vi "Ionospheric image processing ver.1.0 .vi"() -> ()   [LabVIEW 2021]
panel:
  in  "新元素/子数组":i32=1
  out "骨骼化1":dbl[][](graph)
  out "腐蚀":dbl[][](graph)
  out "膨胀":dbl[][](graph)
  out "强度图":dbl[][](graph)
  out "大小":i32[](array[numeric])
  in  "y":i32
  out "x与y？":bool
  out "骨骼化0.5":dbl[][](graph)
  in  "dy":dbl=2.5 format="%#_13g"
  in  "y_max":dbl=900.0 format="%#_13g"
  in  "y_min":dbl format="%#_13g"
  in  "dx":dbl=0.05 format="%#_13g"
  in  "x_max":dbl=10.0 format="%#_13g"
  in  "x_min":dbl=1.5 format="%#_13g"
  in  "路径":path
  # "x:1.5-10\ny:0-900\ndx:0.05\ndy:2.5"
  # "每个x对应多个y值，取中位数或平均值，同时参考x前的值或x后的值，使得曲线变得更加平滑\n（需了解相关函数）"
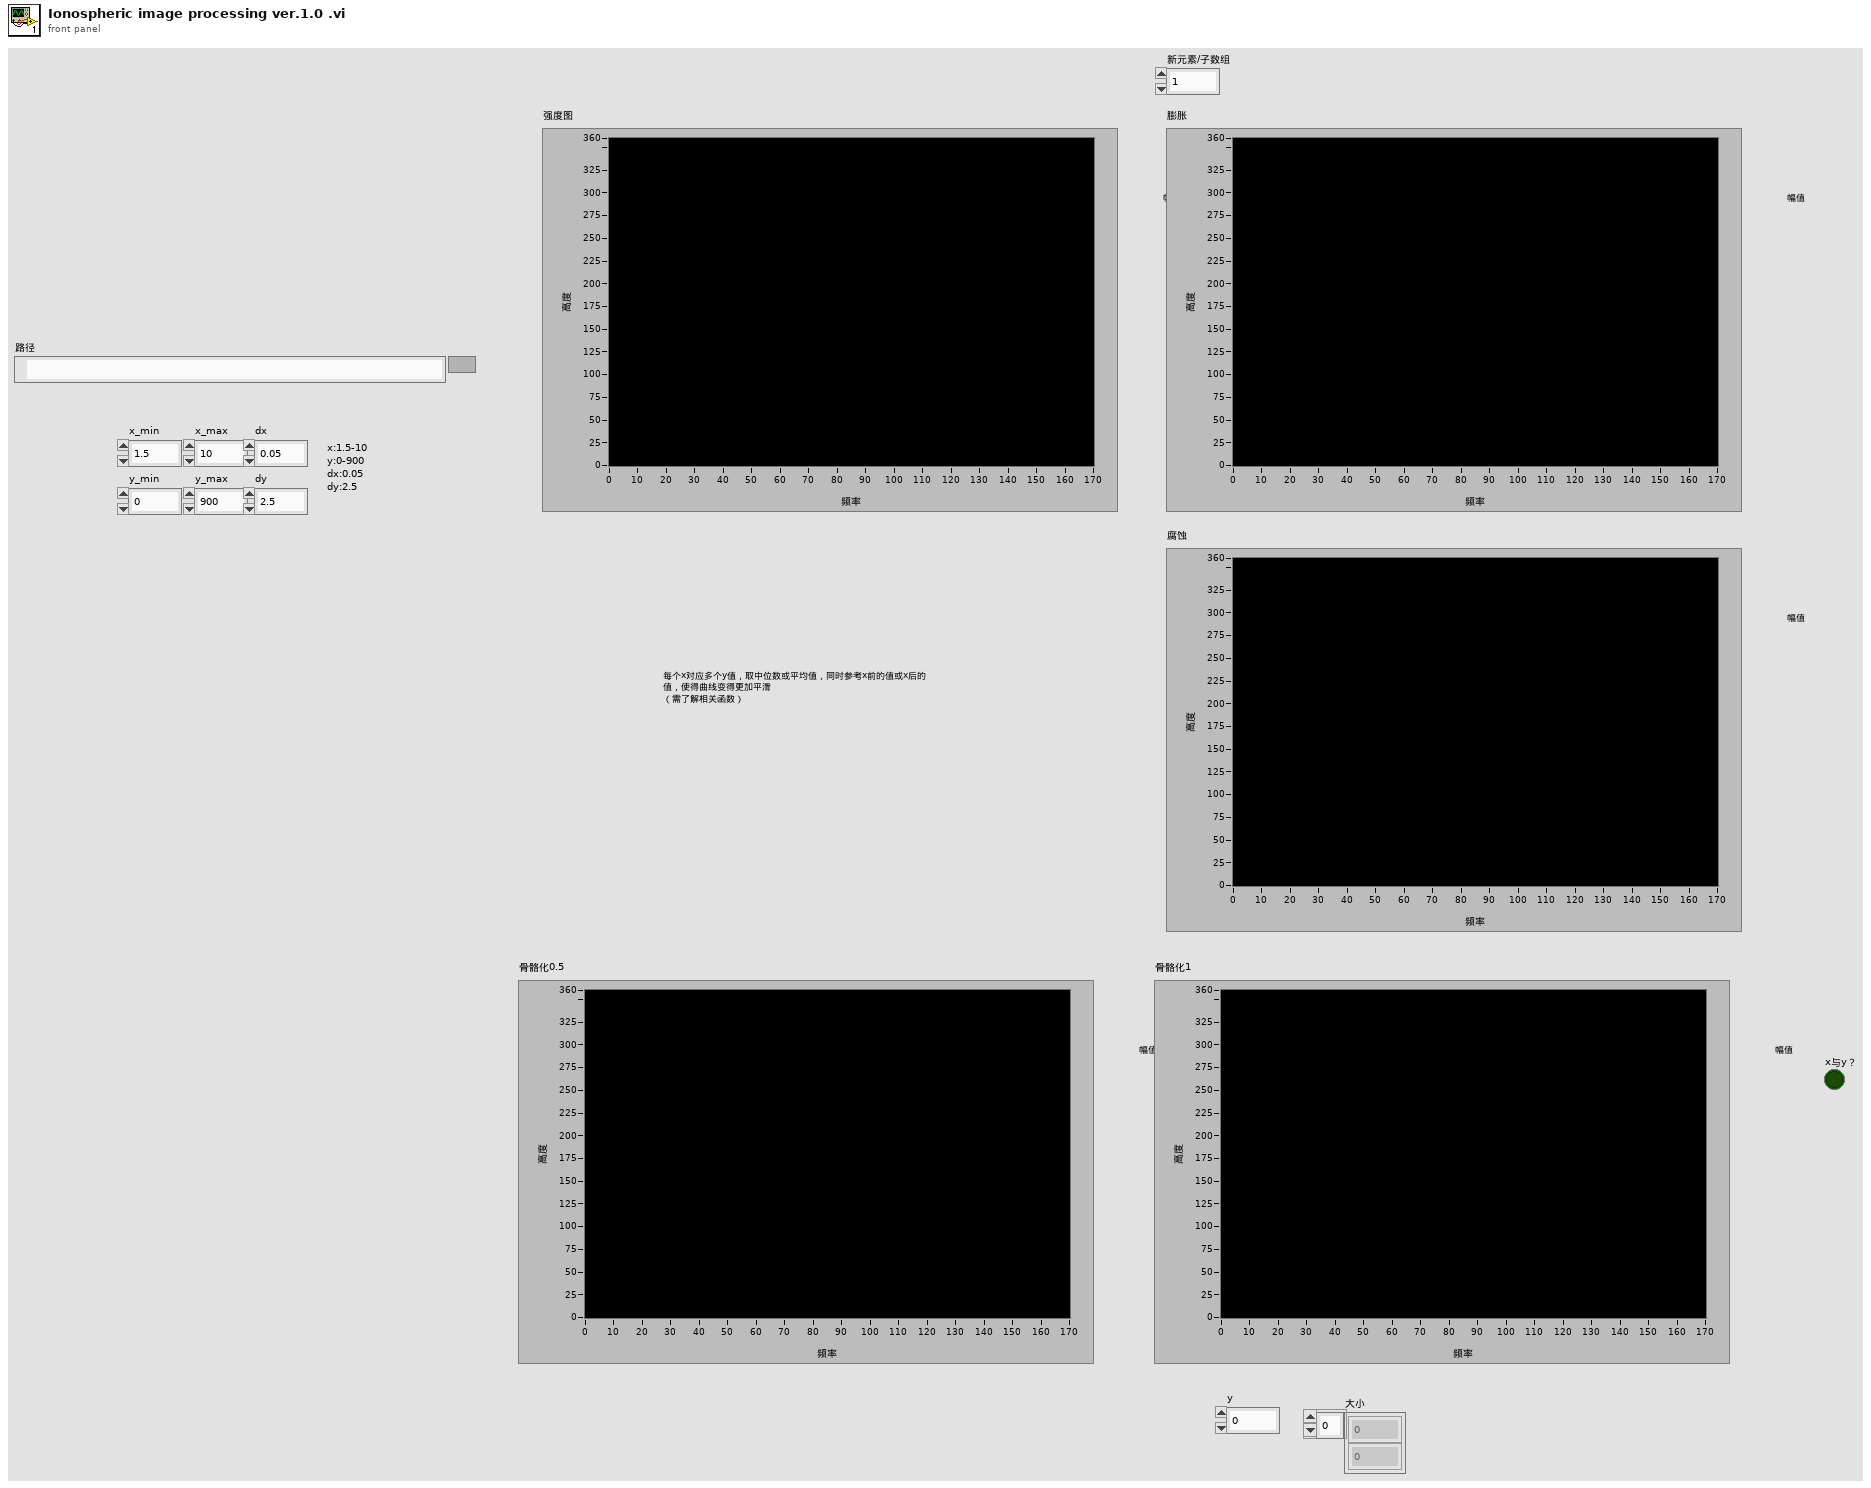
[diagram p1: front panel]
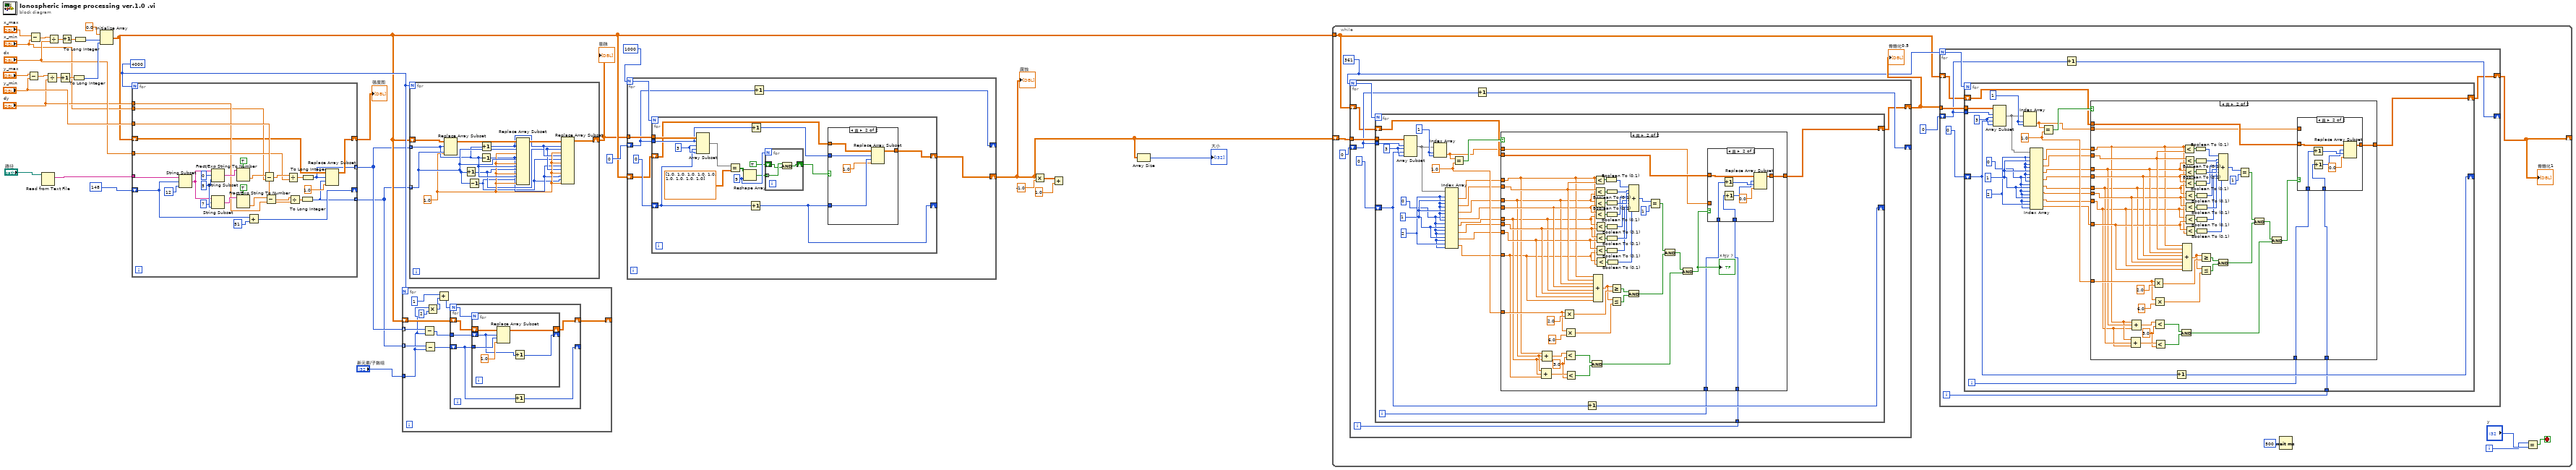
[diagram p0: block diagram]
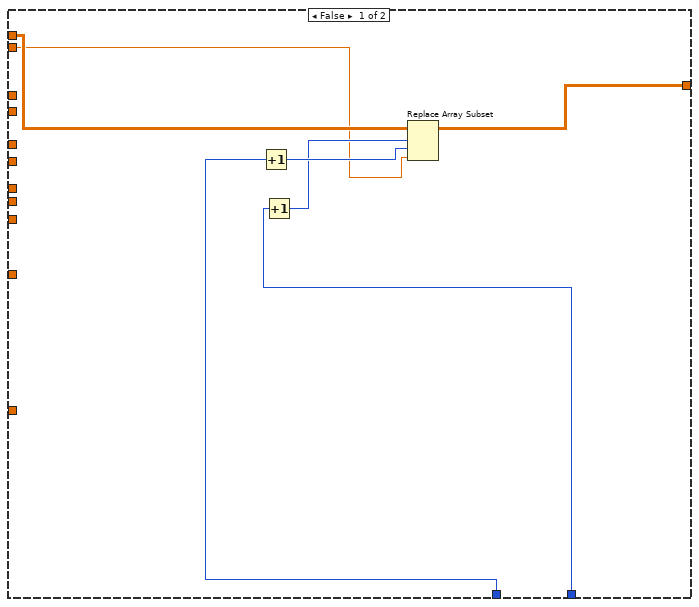
[diagram p2: hidden frame]
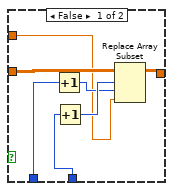
[diagram p3: hidden frame]
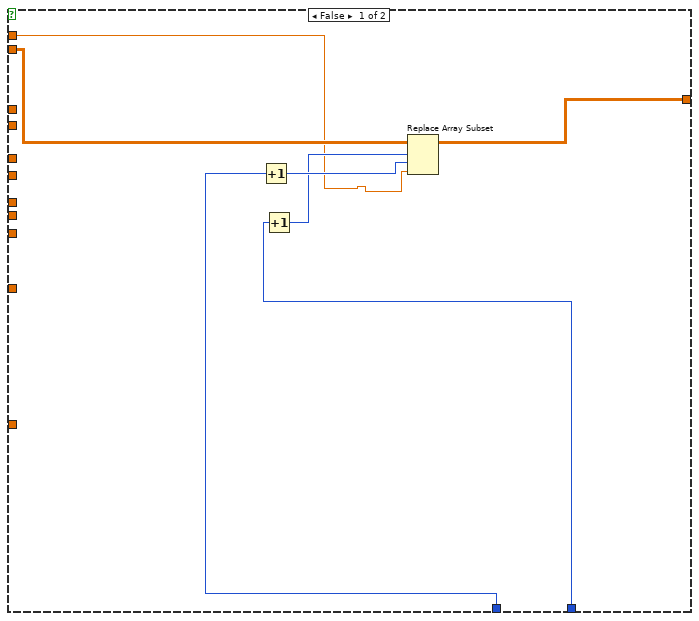
[diagram p4: hidden frame]
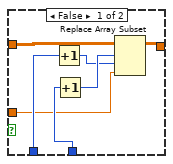
[diagram p5: hidden frame]
diagram:
  w5 = 4000
  n1 = Subtract(x="y_max", y="y_min") -> (x-y=w27:dbl)
  n2 = Subtract(x="x_max", y="x_min") -> (x-y=w31:dbl)
  n3 = Read from Text File(file (use dialog)="路径") -> (text=w20:string)  [unwired: 3 in, 3 out]
  n4 = Divide(x=w27, y="dy") -> (x/y=w26:dbl)
  n5 = Divide(x=w31, y="dx") -> (x/y=w30:dbl)
  n6 = Increment(x=w26) -> (x+1=w25:dbl)
  n7 = Increment(x=w30) -> (x+1=w29:dbl)
  n8 = To Long Integer(number=w25) -> (32bit integer=w22:i32)
  n9 = To Long Integer(number=w29) -> (32bit integer=w28:i32)
  n10 = Initialize Array(0.0 ("元素"), w28, w22) -> (w4:dbl[][])
  n11 = for {
    N: w5 -> [_]
    tunnel: w20 -> [w60]
    tunnel: "y_min" -> [w47]
    tunnel: "dx" -> [w45]
    tunnel: "dy" -> [w43]
    tunnel: "x_min" -> [w39]
    shift-right: [w38] -> w8
    shift-left: w4 -> [w37]
    shift-right: [w36] -> _
    shift-left: 148 ("偏移量(0)") -> [w35]
    tunnel: [w34] -> w3 mode=indexing
    tunnel: [w33] -> w2 mode=indexing
    w57 = 5 ("长度（剩余）")
    n12 = String Subset(string=w60, offset (0)=w35, length (rest)=12 ("长度（剩余）")) -> (substring=w56:string)
    n13 = String Subset(string=w56, offset (0)=0 ("偏移量(0)"), length (rest)=w57) -> (substring=w52:string)
    n14 = String Subset(string=w56, offset (0)=7 ("偏移量(0)"), length (rest)=w57) -> (substring=w50:string)
    n15 = Fract/Exp String To Number(use system decimal point (T)=TRUE ("使用系统小数点(T)"), string=w52) -> (number=w49:dbl)  [unwired: 2 in, 1 out]
    n16 = Fract/Exp String To Number(use system decimal point (T)=TRUE ("使用系统小数点(T)"), string=w50) -> (number=w48:dbl)  [unwired: 2 in, 1 out]
    n17 = Add(x=w35, y=51) -> (x+y=w36:i32)
    n18 = Subtract(x=w49, y=w39) -> (x-y=w46:dbl)
    n19 = Subtract(x=w48, y=w47) -> (x-y=w44:dbl)
    n20 = Divide(x=w46, y=w45) -> (x/y=w42:dbl)
    n21 = Divide(x=w44, y=w43) -> (x/y=w41:dbl)
    n22 = To Long Integer(number=w41) -> (32bit integer=w33:i32)
    n23 = To Long Integer(number=w42) -> (32bit integer=w34:i32)
    n24 = Replace Array Subset(array=w37, new element=1.0 ("元素"), index (row)=w34, index (col)=w33) -> (w38:dbl[][])
  }
  "强度图" <- w8
  n25 = for {
    N: w5 -> [_]
    tunnel: "新元素/子数组" -> [w66]
    tunnel: w3 -> [w70] mode=indexing
    tunnel: w2 -> [w69] mode=indexing
    shift-right: [w61] -> _
    shift-left: w4 -> [w71]
    n26 = Subtract(x=w70, y=w66) -> (x-y=w63:i32)
    n27 = Subtract(x=w69, y=w66) -> (x-y=w62:i32)
    n28 = Multiply(x=w66, y=2) -> (x*y=w67:i32)
    n29 = Add(x=1 ("新元素/子数组"), y=w67) -> (x+y=w64:i32)
    n30 = for {
      N: w64 -> [w76]
      shift-right: [w74] -> w61
      shift-left: w71 -> [w77]
      tunnel: w63 -> [w75]
      shift-right: [w73] -> _
      shift-left: w62 -> [w72]
      n31 = for {
        N: w76 -> [_]
        shift-right: [w80] -> w74
        shift-left: w77 -> [w83]
        tunnel: w72 -> [w81]
        shift-right: [w78] -> _
        shift-left: w75 -> [w79]
        n32 = Replace Array Subset(array=w83, new element=1.0 ("新元素/子数组"), index (row)=w79, index (col)=w81) -> (w80:dbl[][])
        n33 = Increment(x=w79) -> (x+1=w78:i32)
      }
      n34 = Increment(x=w72) -> (x+1=w73:i32)
    }
  }
  n35 = for {
    N: w5 -> [_]
    shift-right: [w84] -> w1
    shift-left: w4 -> [w94]
    tunnel: w3 -> [w91] mode=indexing
    tunnel: w2 -> [w92] mode=indexing
    w89 = 1.0 ("新元素/子数组")
    n36 = Replace Array Subset(array=w94, new element=w89, index (row)=w91, index (col)=w92) -> (w93:dbl[][])
    n37 = Increment(x=w92) -> (x+1=w87:i32)
    n38 = Decrement(x=w92) -> (x-1=w85:i32)
    n39 = Decrement(x=w91) -> (x-1=w86:i32)
    n40 = Increment(x=w91) -> (x+1=w88:i32)
    n41 = Replace Array Subset(array=w93, new element #1=w89, index (row) #1=w88, index (col) #1=w92, new element #2=w89, index (row) #2=w86, index (col) #2=w92, new element #3=w89, index (row) #3=w91, index (col) #3=w87, new element #4=w89, index (row) #4=w91, index (col) #4=w85) -> (w90:dbl[][])
    n42 = Replace Array Subset(array=w90, new element #1=w89, index (row) #1=w88, index (col) #1=w87, new element #2=w89, index (row) #2=w88, index (col) #2=w85, new element #3=w89, index (row) #3=w86, index (col) #3=w87, new element #4=w89, index (row) #4=w86, index (col) #4=w85) -> (w84:dbl[][])
  }
  "膨胀" <- w1
  n43 = for {
    N: 1000 ("数值") -> [w100]
    tunnel: w1 -> [w101]
    shift-right: [w98] -> _
    shift-left: 0 ("索引") -> [w99]
    shift-right: [w96] -> w7
    shift-left: w4 -> [w95]
    n44 = for {
      N: w100 -> [_]
      tunnel: w101 -> [w116]
      tunnel: w99 -> [w106]
      shift-right: [w104] -> _
      shift-left: 0 ("索引") -> [w105]
      shift-right: [w103] -> w96
      shift-left: w95 -> [w102]
      w112 = 9 ("维数大小")
      w115 = 3 ("长度")
      n45 = Array Subset(array=w116, index (row)=w106, length (row)=w115, index (col)=w105, length (col)=w115) -> (w108:dbl[][])
      n46 = Equal?(x=w108, y=dbl[][] [[1.0, 1.0, 1.0], [1.0, 1.0, 1.0], [1.0, 1.0, 1.0]]) -> (x = y?=w113:bool[][])
      n47 = Reshape Array(w113, w112) -> (w111:bool[])
      n48 = Increment(x=w105) -> (x+1=w104:i32)
      n49 = Increment(x=w106) -> (x+1=w107:i32)
      n50 = for {
        N: w112 -> [_]
        shift-right: [w123] -> w109
        shift-left: TRUE -> [w124]
        tunnel: w111 -> [w125] mode=indexing
        n51 = And(x=w125, y=w124) -> (x .and. y?=w123:bool)
      }
      n52 = case shown="真" w109 {
        tunnel: w102 -> [w117 w122]
        tunnel: [w117 w121] -> w103
        tunnel: w107 -> [_ w120]
        tunnel: w104 -> [_ w119]
        frame False {
        }
        frame True {
          n53 = Replace Array Subset(array=w122, new element=1.0 ("新元素/子数组"), index (row)=w120, index (col)=w119) -> (w121:dbl[][])
        }
      }
    }
    n54 = Increment(x=w99) -> (x+1=w98:i32)
  }
  "腐蚀" <- w7
  n55 = Multiply(x=w7, y=-1.0) -> (x*y=w11:dbl[][])
  n56 = Add(x=w11, y=1.0) -> ()  [unwired: 1 out]
  n57 = Array Size(array=w7) -> (size(s)=→"大小":i32[])
  n58 = while {
    tunnel: w4 -> [w132]
    shift-right: [w128] -> _
    shift-left: w7 -> [w136]
    i -> [w127]
    stop <- w130 stop-if-true
    w133 = 361
    n59 = for {
      N: w133 -> [w246]
      tunnel: w136 -> [w247]
      shift-right: [w244] -> _
      shift-left: 0 ("索引") -> [w245]
      shift-right: [w240] -> w134
      shift-left: w132 -> [w241]
      i -> [w242]
      n60 = for {
        N: w246 -> [_]
        tunnel: w247 -> [w272]
        tunnel: w245 -> [w270]
        shift-right: [w265] -> _
        shift-left: 0 ("索引") -> [w266]
        tunnel: w242 -> [w263]
        shift-right: [w261] -> w240
        shift-left: w241 -> [w262]
        i -> [w264]
        w250 = 2
        w251 = 1
        w249 = 0
        w267 = 1.0 ("新元素/子数组")
        w268 = 1 ("长度")
        w271 = 3 ("长度")
        n61 = Array Subset(array=w272, index (row)=w270, length (row)=w271, index (col)=w266, length (col)=w271) -> (w260:dbl[][])
        n62 = Index Array(array=w260, index (row)=w268, index (col)=w268) -> (element=w248:dbl)
        n63 = Index Array(array=w260, index (row) #1=w250, index (col) #1=w251, index (row) #2=w250, index (col) #2=w250, index (row) #3=w251, index (col) #3=w250, index (row) #4=w249, index (col) #4=w250, index (row) #5=w249, index (col) #5=w251, index (row) #6=w249, index (col) #6=w249, index (row) #7=w251, index (col) #7=w249, index (row) #8=w250, index (col) #8=w249) -> (element #1=w259:dbl, element #2=w258:dbl, element #3=w257:dbl, element #4=w256:dbl, element #5=w255:dbl, element #6=w254:dbl, element #7=w253:dbl, element #8=w252:dbl)
        n64 = Equal?(x=w248, y=w267) -> (x = y?=w269:bool)
        n65 = case shown="真" w269 {
          tunnel: w259 -> [_ w298]
          tunnel: w258 -> [_ w310]
          tunnel: w257 -> [_ w297]
          tunnel: w256 -> [_ w309]
          tunnel: w255 -> [_ w296]
          tunnel: w254 -> [_ w308]
          tunnel: w253 -> [_ w307]
          tunnel: w252 -> [_ w295]
          tunnel: w267 -> [_ w304]
          tunnel: [w279 w284] -> w261
          tunnel: w264 -> [w278 w283]
          tunnel: w263 -> [w275 w282]
          tunnel: w262 -> [w274 w281]
          tunnel: w248 -> [w273 w280]
          frame False {
            n66 = Increment(x=w278) -> (x+1=w277:i32)
            n67 = Increment(x=w275) -> (x+1=w276:i32)
            n68 = Replace Array Subset(array=w274, new element=w273, index (row)=w276, index (col)=w277) -> (w279:dbl[][])
          }
          frame True {
            w292 = 3.0 ("y")
            n69 = Compound Arithmetic op=ADD ("复合运算")(w297, w296, w295) -> (w293:dbl)
            n70 = Compound Arithmetic op=ADD ("复合运算")(w298, w297, w296) -> (w294:dbl)
            n71 = Multiply(x=w304, y=2.0) -> (x*y=w303:dbl)
            n72 = Multiply(x=w304, y=6.0) -> (x*y=w302:dbl)
            n73 = Less?(x=w294, y=w292) -> (x < y?=w291:bool)
            n74 = Less?(x=w293, y=w292) -> (x < y?=w290:bool)
            n75 = And(x=w291, y=w290) -> (x .and. y?=w286:bool)
            n76 = Compound Arithmetic op=ADD ("复合运算")(w298, w310, w297, w309, w296, w308, w307, w295) -> (w301:dbl)
            n77 = Less?(x=w298, y=w310) -> (x < y?=w328:bool)
            n78 = Less?(x=w310, y=w297) -> (x < y?=w327:bool)
            n79 = Less?(x=w297, y=w309) -> (x < y?=w326:bool)
            n80 = Less?(x=w309, y=w296) -> (x < y?=w325:bool)
            n81 = Less?(x=w296, y=w308) -> (x < y?=w324:bool)
            n82 = Less?(x=w308, y=w307) -> (x < y?=w323:bool)
            n83 = Less?(x=w307, y=w295) -> (x < y?=w322:bool)
            n84 = Less?(x=w295, y=w298) -> (x < y?=w321:bool)
            n85 = Boolean To (0,1)(Boolean=w328) -> (0, 1=w320:i16)
            n86 = Boolean To (0,1)(Boolean=w327) -> (0, 1=w319:i16)
            n87 = Boolean To (0,1)(Boolean=w326) -> (0, 1=w318:i16)
            n88 = Boolean To (0,1)(Boolean=w325) -> (0, 1=w317:i16)
            n89 = Boolean To (0,1)(Boolean=w324) -> (0, 1=w316:i16)
            n90 = Boolean To (0,1)(Boolean=w323) -> (0, 1=w315:i16)
            n91 = Boolean To (0,1)(Boolean=w322) -> (0, 1=w314:i16)
            n92 = Boolean To (0,1)(Boolean=w321) -> (0, 1=w313:i16)
            n93 = Greater Or Equal?(x=w301, y=w303) -> (x >= y?=w300:bool)
            n94 = Less Or Equal?(x=w301, y=w302) -> (x <= y?=w299:bool)
            n95 = And(x=w300, y=w299) -> (x .and. y?=w288:bool)
            n96 = Compound Arithmetic op=ADD ("复合运算")(w320, w319, w318, w317, w316, w315, w314, w313) -> (w312:i16)
            n97 = Equal?(x=w312, y=i16 1) -> (x = y?=w289:bool)
            n98 = And(x=w289, y=w288) -> (x .and. y?=w287:bool)
            n99 = And(x=w287, y=w286) -> (x .and. y?=w285:bool)
            "x与y？" <- w285
            n100 = case shown="真" w285 {
              tunnel: w281 -> [w335 w342]
              tunnel: [w334 w340] -> w284
              tunnel: w283 -> [w333 w339]
              tunnel: w282 -> [w332 w338]
              tunnel: w280 -> [w329 _]
              frame False {
                n101 = Increment(x=w333) -> (x+1=w330:i32)
                n102 = Increment(x=w332) -> (x+1=w331:i32)
                n103 = Replace Array Subset(array=w335, new element=w329, index (row)=w331, index (col)=w330) -> (w334:dbl[][])
              }
              frame True {
                n104 = Increment(x=w339) -> (x+1=w337:i32)
                n105 = Increment(x=w338) -> (x+1=w336:i32)
                n106 = Replace Array Subset(array=w342, new element=0.0 ("新元素/子数组"), index (row)=w336, index (col)=w337) -> (w340:dbl[][])
              }
            }
          }
        }
        n107 = Increment(x=w266) -> (x+1=w265:i32)
      }
      n108 = Increment(x=w245) -> (x+1=w244:i32)
    }
    "骨骼化0.5" <- w134
    n109 = for {
      N: w133 -> [w143]
      tunnel: w134 -> [w144]
      shift-right: [w141] -> _
      shift-left: 0 ("索引") -> [w142]
      shift-right: [w137] -> w128
      shift-left: w132 -> [w138]
      i -> [w139]
      n110 = for {
        N: w143 -> [_]
        tunnel: w144 -> [w169]
        tunnel: w142 -> [w167]
        shift-right: [w163] -> _
        shift-left: 0 ("索引") -> [w164]
        tunnel: w139 -> [w161]
        shift-right: [w159] -> w137
        shift-left: w138 -> [w160]
        i -> [w162]
        w156 = 2
        w157 = 1
        w155 = 0
        w158 = 1.0 ("新元素/子数组")
        w165 = 1 ("长度")
        w168 = 3 ("长度")
        n111 = Array Subset(array=w169, index (row)=w167, length (row)=w168, index (col)=w164, length (col)=w168) -> (w154:dbl[][])
        n112 = Index Array(array=w154, index (row)=w165, index (col)=w165) -> (element=w145:dbl)
        n113 = Index Array(array=w154, index (row) #1=w156, index (col) #1=w157, index (row) #2=w156, index (col) #2=w156, index (row) #3=w157, index (col) #3=w156, index (row) #4=w155, index (col) #4=w156, index (row) #5=w155, index (col) #5=w157, index (row) #6=w155, index (col) #6=w155, index (row) #7=w157, index (col) #7=w155, index (row) #8=w156, index (col) #8=w155) -> (element #1=w153:dbl, element #2=w152:dbl, element #3=w151:dbl, element #4=w150:dbl, element #5=w149:dbl, element #6=w148:dbl, element #7=w147:dbl, element #8=w146:dbl)
        n114 = Equal?(x=w145, y=w158) -> (x = y?=w166:bool)
        n115 = case shown="真" w166 {
          tunnel: w153 -> [_ w180]
          tunnel: w152 -> [_ w207]
          tunnel: w151 -> [_ w181]
          tunnel: w150 -> [_ w206]
          tunnel: w149 -> [_ w179]
          tunnel: w148 -> [_ w205]
          tunnel: w147 -> [_ w178]
          tunnel: w146 -> [_ w182]
          tunnel: w158 -> [_ w202]
          tunnel: [w176 w186] -> w159
          tunnel: w162 -> [w175 w185]
          tunnel: w161 -> [w172 w184]
          tunnel: w160 -> [w171 w183]
          tunnel: w145 -> [w170 w177]
          frame False {
            n116 = Increment(x=w175) -> (x+1=w174:i32)
            n117 = Increment(x=w172) -> (x+1=w173:i32)
            n118 = Replace Array Subset(array=w171, new element=w170, index (row)=w173, index (col)=w174) -> (w176:dbl[][])
          }
          frame True {
            w194 = 3.0 ("y")
            n119 = Compound Arithmetic op=ADD ("复合运算")(w180, w179, w178) -> (w195:dbl)
            n120 = Compound Arithmetic op=ADD ("复合运算")(w180, w181, w178) -> (w196:dbl)
            n121 = Multiply(x=w202, y=2.0) -> (x*y=w201:dbl)
            n122 = Multiply(x=w202, y=6.0) -> (x*y=w200:dbl)
            n123 = Less?(x=w196, y=w194) -> (x < y?=w193:bool)
            n124 = Less?(x=w195, y=w194) -> (x < y?=w192:bool)
            n125 = And(x=w193, y=w192) -> (x .and. y?=w188:bool)
            n126 = Compound Arithmetic op=ADD ("复合运算")(w180, w207, w181, w206, w179, w205, w178, w182) -> (w199:dbl)
            n127 = Less?(x=w180, y=w207) -> (x < y?=w225:bool)
            n128 = Less?(x=w207, y=w181) -> (x < y?=w224:bool)
            n129 = Less?(x=w181, y=w206) -> (x < y?=w223:bool)
            n130 = Less?(x=w206, y=w179) -> (x < y?=w222:bool)
            n131 = Less?(x=w179, y=w205) -> (x < y?=w221:bool)
            n132 = Less?(x=w205, y=w178) -> (x < y?=w220:bool)
            n133 = Less?(x=w178, y=w182) -> (x < y?=w219:bool)
            n134 = Less?(x=w182, y=w180) -> (x < y?=w218:bool)
            n135 = Boolean To (0,1)(Boolean=w225) -> (0, 1=w217:i16)
            n136 = Boolean To (0,1)(Boolean=w224) -> (0, 1=w216:i16)
            n137 = Boolean To (0,1)(Boolean=w223) -> (0, 1=w215:i16)
            n138 = Boolean To (0,1)(Boolean=w222) -> (0, 1=w214:i16)
            n139 = Boolean To (0,1)(Boolean=w221) -> (0, 1=w213:i16)
            n140 = Boolean To (0,1)(Boolean=w220) -> (0, 1=w212:i16)
            n141 = Boolean To (0,1)(Boolean=w219) -> (0, 1=w211:i16)
            n142 = Boolean To (0,1)(Boolean=w218) -> (0, 1=w210:i16)
            n143 = Greater Or Equal?(x=w199, y=w201) -> (x >= y?=w198:bool)
            n144 = Less Or Equal?(x=w199, y=w200) -> (x <= y?=w197:bool)
            n145 = And(x=w198, y=w197) -> (x .and. y?=w190:bool)
            n146 = Compound Arithmetic op=ADD ("复合运算")(w217, w216, w215, w214, w213, w212, w211, w210) -> (w209:i16)
            n147 = Equal?(x=w209, y=i16 1) -> (x = y?=w191:bool)
            n148 = And(x=w191, y=w190) -> (x .and. y?=w189:bool)
            n149 = And(x=w189, y=w188) -> (x .and. y?=w187:bool)
            n150 = case shown="真" w187 {
              tunnel: w183 -> [w232 w239]
              tunnel: [w231 w237] -> w186
              tunnel: w185 -> [w230 w236]
              tunnel: w184 -> [w229 w235]
              tunnel: w177 -> [w226 _]
              frame False {
                n151 = Increment(x=w230) -> (x+1=w227:i32)
                n152 = Increment(x=w229) -> (x+1=w228:i32)
                n153 = Replace Array Subset(array=w232, new element=w226, index (row)=w228, index (col)=w227) -> (w231:dbl[][])
              }
              frame True {
                n154 = Increment(x=w236) -> (x+1=w234:i32)
                n155 = Increment(x=w235) -> (x+1=w233:i32)
                n156 = Replace Array Subset(array=w239, new element=0.0 ("新元素/子数组"), index (row)=w233, index (col)=w234) -> (w237:dbl[][])
              }
            }
          }
        }
        n157 = Increment(x=w164) -> (x+1=w163:i32)
      }
      n158 = Increment(x=w142) -> (x+1=w141:i32)
    }
    "骨骼化1" <- w128
    n159 = Wait (ms)(milliseconds to wait=u32 500 ("等待时间（毫秒）")) -> ()  [unwired: 1 out]
    n160 = Equal?(x=w127, y="y") -> (x = y?=w130:bool)
  }
